vi "Initialize Sensors and Pnuematics.vi"   [LabVIEW 2017]
uses:
  <vilib>/Rock Robotics/SystemInterfaces/AI/FPGA_AIChannel.ctl
  <vilib>/Rock Robotics/SystemInterfaces/DIO/FPGA_DIOChannel.ctl
  <vilib>/Rock Robotics/WPI/Encoder/WPI_EncoderType.ctl
  <vilib>/Rock Robotics/WPI/Solenoid/WPI_SolenoidChannel.ctl
  <vilib>/Rock Robotics/WPI/Utilities/WPI_GetSetVariantRefNum.vi
  Globals/Robot Global Data.vi
  <vilib>/Rock Robotics/WPI/Counter/WPI_CounterDigitalInputToDigitalSource.vi
  <vilib>/Rock Robotics/WPI/Solenoid/WPI_SolenoidOpenSingle.vi
  <vilib>/Rock Robotics/WPI/Switch/WPI_SwitchOpenLimit.vi
types:
  T1 = typedef "WPI_SolenoidChannel.ctl" = enum8{"Solenoid 0", "Solenoid 1", "Solenoid 2", "Solenoid 3", "Solenoid 4", "Solenoid 5", "Solenoid 6", "Solenoid 7", "Invalid"}
  T2 = typedef "WPI_SolenoidDevRef.ctl" = cluster{"DevStatus":errorcluster, "Pneumatics Control Module":u8, "Forward Solenoid Channel":T1, "Reverse Solenoid Channel":T1}
  T3 = typedef "FPGA_DIOChannel.ctl" = enum8{"DIO 0", "DIO 1", "DIO 2", "DIO 3", "DIO 4", "DIO 5", "DIO 6", "DIO 7", "DIO 8", "DIO 9", "DIO MXP 0", "DIO MXP 1", "DIO MXP 2", "DIO MXP 3", "DIO MXP 4", "DIO MXP 5", "DIO MXP 6", "DIO MXP 7", "DIO MXP 8", "DIO MXP 9", "DIO MXP 10", "DIO MXP 11", "DIO MXP 12", "DIO MXP 13", "DIO MXP 14", "DIO MXP 15", "SPI Port CS1", "SPI Port CS2", "SPI Port CS3", "SPI Port MISO", "SPI Port MOSI", "Invalid"}
  T4 = typedef "WPI_EncoderType.ctl" = enum16{"1x", "2x", "4x"}
  T5 = typedef "WPI_DigitalInputDevRef.ctl" = cluster{"DevStatus":errorcluster, "DIO Channel":T3}
  T6 = typedef "FPGA_CounterEncoderSourceConvertionLVSourceType.ctl" = cluster{"DevStatus":errorcluster, "AnalogTriggerMode?":bool, "DigitalMode":cluster{"DIO Channel":T7}, "AnalogTriggerMode":cluster{"AnalogTriggerIndex":T8, "OutputType":T9}}
  T7 = typedef "FPGA_DIODigitalSourceChannel.ctl" = enum8{"DIO 0", "DIO 1", "DIO 2", "DIO 3", "DIO 4", "DIO 5", "DIO 6", "DIO 7", "DIO 8", "DIO 9", "DIO MXP 0", "DIO MXP 1", "DIO MXP 2", "DIO MXP 3", "DIO MXP 4", "DIO MXP 5", "DIO MXP 6", "DIO MXP 7", "DIO MXP 8", "DIO MXP 9", "DIO MXP 10", "DIO MXP 11", "DIO MXP 12", "DIO MXP 13", "DIO MXP 14", "DIO MXP 15", "Disabled"}
  T8 = typedef "FPGA_AnalogTriggerIndex.ctl" = enum8{"Trig 0", "Trig 1", "Trig 2", "Trig 3", "Trig 4", "Trig 5", "Trig 6", "Trig 7", "Invalid"}
  T9 = typedef "FPGA_AnalogTriggerOutType.ctl" = enum16{"InWindow", "TriggerState", "Rising", "Falling"}
  T10 = typedef "WPI_EncoderDevRef.ctl" = cluster{"DevStatus":errorcluster, "EncoderIndex":T11, "CounterIndex":T12, "DistancePerCount":dbl, "Decoding Type":T4}
  T11 = typedef "FPGA_EncoderIdx.ctl" = enum8{"Enc 0", "Enc 1", "Enc 2", "Enc 3", "Enc 4", "Enc 5", "Enc 6", "Enc 7", "Invalid"}
  T12 = typedef "FPGA_CounterCtrSystemIndex.ctl" = enum8{"Ctr 0", "Ctr 1", "Ctr 2", "Ctr 3", "Ctr 4", "Ctr 5", "Ctr 6", "Ctr 7", "Invalid"}
  T13 = typedef "WPI_CompressorDevRef.ctl" = cluster{"DevStatus":errorcluster, "Pneumatics Control Module":u8}
  T14 = typedef "FPGA_AIChannel.ctl" = enum8{"AI 0", "AI 1", "AI 2", "AI 3", "AI MXP 0", "AI MXP 1", "AI MXP 2", "AI MXP 3", "Invalid"}
  T15 = typedef "WPI_AnalogChannelDevRef.ctl" = cluster{"DevStatus":errorcluster, "Analog Channel":T14}
  T16 = typedef "WPI_SwitchDevRef.ctl" = cluster{"DevStatus":errorcluster, "DIO Channel":T3, "CntIndex":T12, "Normally Closed":bool}
  T17 = typedef "WPI_PotentiometerDevRef.ctl" = cluster{"DevStatus":errorcluster, "Analog Channel":T14, "Invert Output":bool}
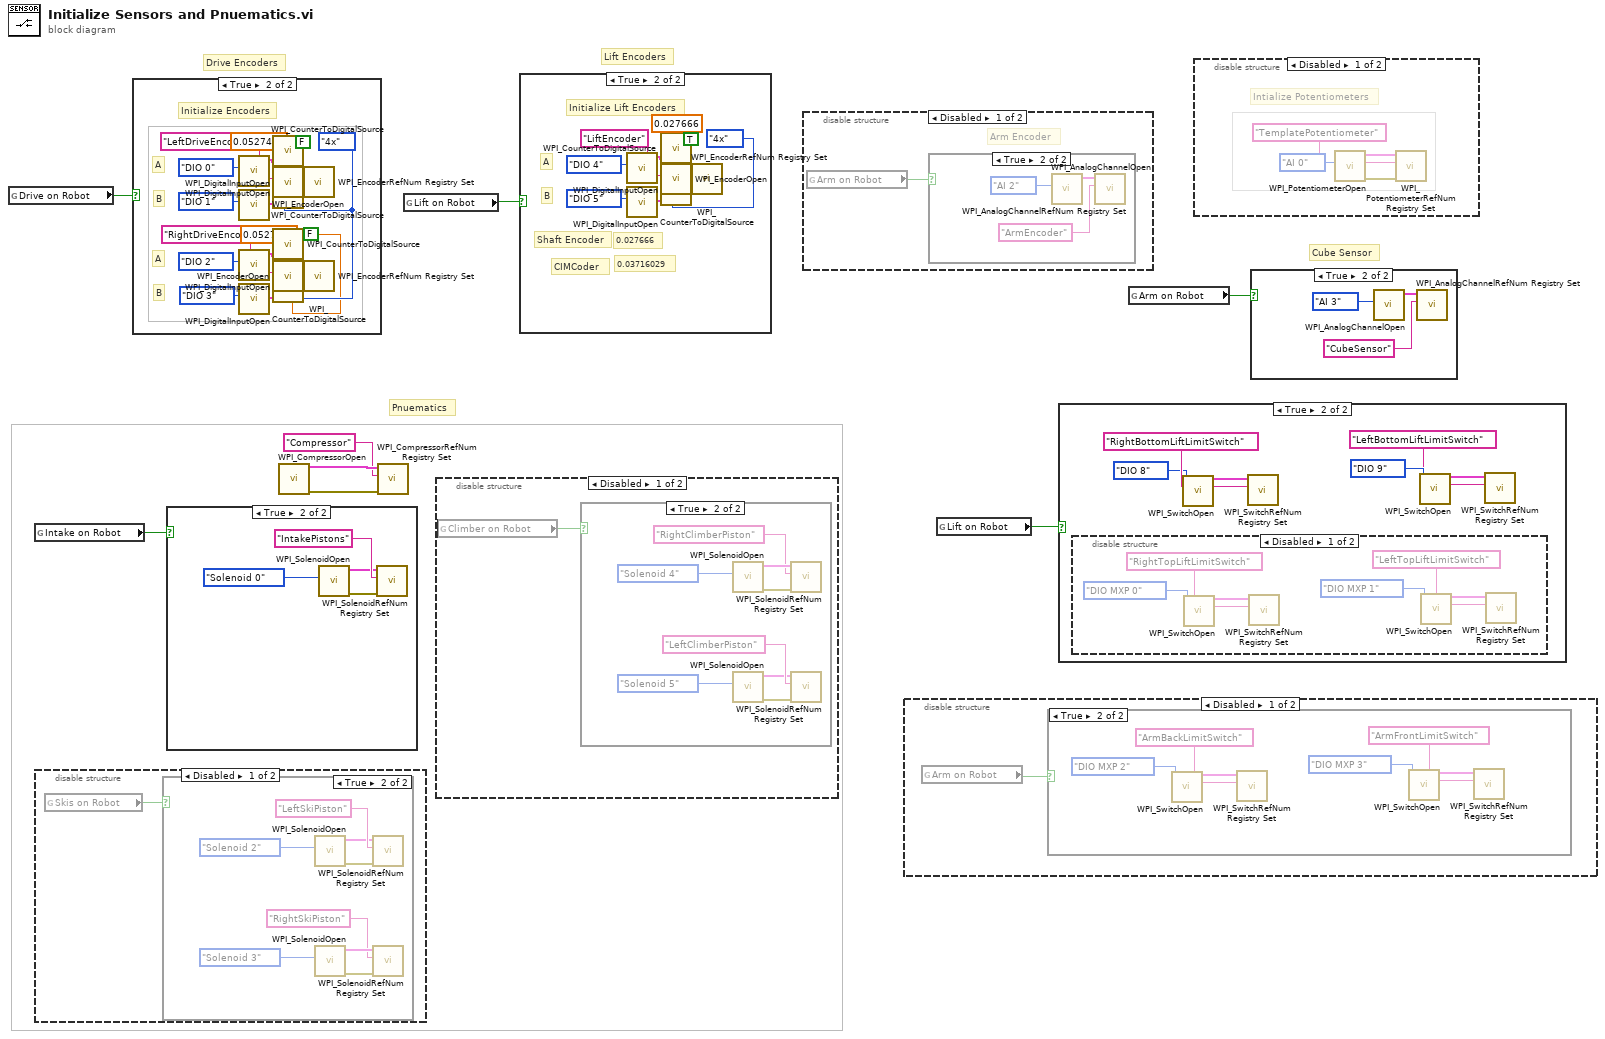
[diagram p0: block diagram]
diagram:
  # "Cube Sensor"
  # "Lift Encoders"
  # "Drive Encoders"
  # "Pnuematics"
  n1 = global read "Robot Global Data.vi" "Drive on Robot"() -> (w5:bool)
  n2 = global read "Robot Global Data.vi" "Intake on Robot"() -> (w4:bool)
  n3 = disable-structure shown="Disabled" {
    frame Disabled {
      n4 = global read "Robot Global Data.vi" "Skis on Robot"() -> (w9:bool)
      n5 = case shown="True" w9 {
        frame False {
        }
        frame True {
          n6 = call-poly <vilib>:"WPI_SolenoidOpen.vi"("Solenoid Channel"=WPI_SolenoidChannel."Solenoid 2") -> ("error out"=w12:errorcluster, "SolenoidDevRef"=w13:T2)  [unwired: 9 in]
          n7 = call-poly <vilib>:"WPI_SolenoidOpen.vi"("Solenoid Channel"=WPI_SolenoidChannel."Solenoid 3") -> ("error out"=w17:errorcluster, "SolenoidDevRef"=w16:T2)  [unwired: 9 in]
          n8 = call <vilib>:"WPI_SolenoidRefNum Registry Set.vi"("error in (no error)"=w12, "refnum name"="LeftSkiPiston", "SolenoidDevRef"=w13) -> ()  [unwired: 7 in, 2 out]
          n9 = call <vilib>:"WPI_SolenoidRefNum Registry Set.vi"("error in (no error)"=w17, "refnum name"="RightSkiPiston", "SolenoidDevRef"=w16) -> ()  [unwired: 7 in, 2 out]
        }
      }
    }
    frame Enabled {
    }
  }
  n10 = case shown="True" w5 {
    frame False {
    }
    frame True {
      w21 = WPI_EncoderType."4x" ("Decoding Type")
      # "B"
      # "A"
      # "B"
      # "A"
      # "Initialize Encoders"
      n11 = call <vilib>:"WPI_DigitalInputOpen.vi"("DIO Channel"=FPGA_DIOChannel."DIO 0") -> ("DigitalInputDevRef"=w38:T5)  [unwired: 1 in, 9 out]
      n12 = call <vilib>:"WPI_DigitalInputOpen.vi"("DIO Channel"=FPGA_DIOChannel."DIO 1") -> ("DigitalInputDevRef"=w39:T5)  [unwired: 1 in, 9 out]
      n13 = call <vilib>:"WPI_DigitalInputOpen.vi"("DIO Channel"=FPGA_DIOChannel."DIO 2") -> ("DigitalInputDevRef"=w29:T5)  [unwired: 1 in, 9 out]
      n14 = call <vilib>:"WPI_DigitalInputOpen.vi"("DIO Channel"=FPGA_DIOChannel."DIO 3") -> ("DigitalInputDevRef"=w30:T5)  [unwired: 1 in, 9 out]
      n15 = call-poly <vilib>:"WPI_CounterToDigitalSource.vi"("DigitalInputDevRef"=w38) -> ("Digital Source"=w37:T6)  [unwired: 6 out]
      n16 = call-poly <vilib>:"WPI_CounterToDigitalSource.vi"("DigitalInputDevRef"=w39) -> ("Digital Source"=w40:T6)  [unwired: 6 out]
      n17 = call <vilib>:"WPI_EncoderOpen.vi"("DistancePerCount"=0.0527473, "Decoding Type"=w21, "Invert Direction (False)"=FALSE, "BSource"=w40, "ASource"=w37) -> ("error out"=w34:errorcluster, "EncoderDevRef"=w33:T10)  [unwired: 3 in, 2 out]
      n18 = call-poly <vilib>:"WPI_CounterToDigitalSource.vi"("DigitalInputDevRef"=w29) -> ("Digital Source"=w28:T6)  [unwired: 6 out]
      n19 = call-poly <vilib>:"WPI_CounterToDigitalSource.vi"("DigitalInputDevRef"=w30) -> ("Digital Source"=w31:T6)  [unwired: 6 out]
      n20 = call <vilib>:"WPI_EncoderOpen.vi"("DistancePerCount"=0.0527473, "Decoding Type"=w21, "Invert Direction (False)"=FALSE, "BSource"=w31, "ASource"=w28) -> ("error out"=w25:errorcluster, "EncoderDevRef"=w24:T10)  [unwired: 3 in, 2 out]
      n21 = call <vilib>:"WPI_EncoderRefNum Registry Set.vi"("error in (no error)"=w34, "refnum name"="LeftDriveEncoder", "EncoderDevRef"=w33) -> ()  [unwired: 7 in, 2 out]
      n22 = call <vilib>:"WPI_EncoderRefNum Registry Set.vi"("error in (no error)"=w25, "refnum name"="RightDriveEncoder", "EncoderDevRef"=w24) -> ()  [unwired: 7 in, 2 out]
    }
  }
  n23 = case shown="True" w4 {
    frame False {
    }
    frame True {
      n24 = call-poly <vilib>:"WPI_SolenoidOpen.vi"("Solenoid Channel"=WPI_SolenoidChannel."Solenoid 0") -> ("error out"=w42:errorcluster, "SolenoidDevRef"=w43:T2)  [unwired: 9 in]
      n25 = call <vilib>:"WPI_SolenoidRefNum Registry Set.vi"("error in (no error)"=w42, "refnum name"="IntakePistons", "SolenoidDevRef"=w43) -> ()  [unwired: 7 in, 2 out]
    }
  }
  n26 = call <vilib>:"WPI_CompressorOpen.vi"() -> ("CompressorDevRef"=w7:T13, "error out"=w8:errorcluster)  [unwired: 14 in]
  n27 = call <vilib>:"WPI_CompressorRefNum Registry Set.vi"("error in (no error)"=w8, "refnum name"="Compressor", "CompressorDevRef"=w7) -> ()  [unwired: 7 in, 2 out]
  n28 = global read "Robot Global Data.vi" "Lift on Robot"() -> (w3:bool)
  n29 = disable-structure shown="Disabled" {
    frame Disabled {
      n30 = global read "Robot Global Data.vi" "Climber on Robot"() -> (w45:bool)
      n31 = case shown="True" w45 {
        frame False {
        }
        frame True {
          n32 = call-poly <vilib>:"WPI_SolenoidOpen.vi"("Solenoid Channel"=WPI_SolenoidChannel."Solenoid 4") -> ("error out"=w53:errorcluster, "SolenoidDevRef"=w52:T2)  [unwired: 9 in]
          n33 = call-poly <vilib>:"WPI_SolenoidOpen.vi"("Solenoid Channel"=WPI_SolenoidChannel."Solenoid 5") -> ("error out"=w48:errorcluster, "SolenoidDevRef"=w49:T2)  [unwired: 9 in]
          n34 = call <vilib>:"WPI_SolenoidRefNum Registry Set.vi"("error in (no error)"=w53, "refnum name"="RightClimberPiston", "SolenoidDevRef"=w52) -> ()  [unwired: 7 in, 2 out]
          n35 = call <vilib>:"WPI_SolenoidRefNum Registry Set.vi"("error in (no error)"=w48, "refnum name"="LeftClimberPiston", "SolenoidDevRef"=w49) -> ()  [unwired: 7 in, 2 out]
        }
      }
    }
    frame Enabled {
    }
  }
  n36 = case shown="True" w3 {
    frame False {
    }
    frame True {
      # "CIMCoder"
      # "Shaft Encoder"
      # "0.03716029"
      # "0.027666"
      # "B"
      # "A"
      # "Initialize Lift Encoders"
      n37 = call <vilib>:"WPI_DigitalInputOpen.vi"("DIO Channel"=FPGA_DIOChannel."DIO 4") -> ("DigitalInputDevRef"=w63:T5)  [unwired: 1 in, 9 out]
      n38 = call <vilib>:"WPI_DigitalInputOpen.vi"("DIO Channel"=FPGA_DIOChannel."DIO 5") -> ("DigitalInputDevRef"=w64:T5)  [unwired: 1 in, 9 out]
      n39 = call-poly <vilib>:"WPI_CounterToDigitalSource.vi"("DigitalInputDevRef"=w63) -> ("Digital Source"=w62:T6)  [unwired: 6 out]
      n40 = call-poly <vilib>:"WPI_CounterToDigitalSource.vi"("DigitalInputDevRef"=w64) -> ("Digital Source"=w65:T6)  [unwired: 6 out]
      n41 = call <vilib>:"WPI_EncoderOpen.vi"("DistancePerCount"=0.027666, "Decoding Type"=WPI_EncoderType."4x", "Invert Direction (False)"=TRUE, "BSource"=w65, "ASource"=w62) -> ("error out"=w59:errorcluster, "EncoderDevRef"=w58:T10)  [unwired: 3 in, 2 out]
      n42 = call <vilib>:"WPI_EncoderRefNum Registry Set.vi"("error in (no error)"=w59, "refnum name"="LiftEncoder", "EncoderDevRef"=w58) -> ()  [unwired: 7 in, 2 out]
    }
  }
  n43 = disable-structure shown="Disabled" {
    frame Disabled {
      # "Arm Encoder"
      n44 = global read "Robot Global Data.vi" "Arm on Robot"() -> (w66:bool)
      n45 = case shown="True" w66 {
        frame False {
        }
        frame True {
          n46 = call <vilib>:"WPI_AnalogChannelOpen.vi"("Analog Channel"=FPGA_AIChannel."AI 2") -> ("AIDeviceRef"=w68:T15)  [unwired: 9 in, 1 out]
          n47 = call <vilib>:"WPI_AnalogChannelRefNum Registry Set.vi"("refnum name"="ArmEncoder", "AIDeviceRef"=w68) -> ()  [unwired: 8 in, 2 out]
        }
      }
    }
    frame Enabled {
    }
  }
  n48 = disable-structure shown="Disabled" {
    frame Disabled {
      n49 = global read "Robot Global Data.vi" "Arm on Robot"() -> (w70:bool)
      n50 = case shown="True" w70 {
        frame False {
        }
        frame True {
          n51 = call-poly <vilib>:"WPI_SwitchOpen.vi"("DIO Channel"=FPGA_DIOChannel."DIO MXP 2") -> ("SwitchDevRef"=w76:T16)  [unwired: 9 in, 1 out]
          n52 = call <vilib>:"WPI_SwitchRefNum Registry Set.vi"("refnum name"="ArmBackLimitSwitch", "SwitchDevRef"=w76) -> ()  [unwired: 8 in, 2 out]
          n53 = call-poly <vilib>:"WPI_SwitchOpen.vi"("DIO Channel"=FPGA_DIOChannel."DIO MXP 3") -> ("SwitchDevRef"=w71:T16)  [unwired: 9 in, 1 out]
          n54 = call <vilib>:"WPI_SwitchRefNum Registry Set.vi"("refnum name"="ArmFrontLimitSwitch", "SwitchDevRef"=w71) -> ()  [unwired: 8 in, 2 out]
        }
      }
    }
    frame Enabled {
    }
  }
  n55 = global read "Robot Global Data.vi" "Lift on Robot"() -> (w2:bool)
  n56 = case shown="True" w2 {
    frame False {
    }
    frame True {
      n57 = disable-structure shown="Disabled" {
        frame Disabled {
          n58 = call-poly <vilib>:"WPI_SwitchOpen.vi"("DIO Channel"=FPGA_DIOChannel."DIO MXP 0") -> ("SwitchDevRef"=w83:T16)  [unwired: 9 in, 1 out]
          n59 = call <vilib>:"WPI_SwitchRefNum Registry Set.vi"("refnum name"="RightTopLiftLimitSwitch", "SwitchDevRef"=w83) -> ()  [unwired: 8 in, 2 out]
          n60 = call-poly <vilib>:"WPI_SwitchOpen.vi"("DIO Channel"=FPGA_DIOChannel."DIO MXP 1") -> ("SwitchDevRef"=w88:T16)  [unwired: 9 in, 1 out]
          n61 = call <vilib>:"WPI_SwitchRefNum Registry Set.vi"("refnum name"="LeftTopLiftLimitSwitch", "SwitchDevRef"=w88) -> ()  [unwired: 8 in, 2 out]
        }
        frame Enabled {
        }
      }
      n62 = call-poly <vilib>:"WPI_SwitchOpen.vi"("DIO Channel"=FPGA_DIOChannel."DIO 8") -> ("SwitchDevRef"=w82:T16)  [unwired: 9 in, 1 out]
      n63 = call <vilib>:"WPI_SwitchRefNum Registry Set.vi"("refnum name"="RightBottomLiftLimitSwitch", "SwitchDevRef"=w82) -> ()  [unwired: 8 in, 2 out]
      n64 = call-poly <vilib>:"WPI_SwitchOpen.vi"("DIO Channel"=FPGA_DIOChannel."DIO 9") -> ("SwitchDevRef"=w77:T16)  [unwired: 9 in, 1 out]
      n65 = call <vilib>:"WPI_SwitchRefNum Registry Set.vi"("refnum name"="LeftBottomLiftLimitSwitch", "SwitchDevRef"=w77) -> ()  [unwired: 8 in, 2 out]
    }
  }
  n66 = global read "Robot Global Data.vi" "Arm on Robot"() -> (w1:bool)
  n67 = disable-structure shown="Disabled" {
    frame Disabled {
      # "Intialize Potentiometers"
      n68 = call <vilib>:"WPI_PotentiometerOpen.vi"("Analog Channel"=FPGA_AIChannel."AI 0") -> ("error out"=w91:errorcluster, "PotDevRef"=w90:T17)  [unwired: 9 in]
      n69 = call <vilib>:"WPI_PotentiometerRefNum Registry Set.vi"("error in (no error)"=w91, "refnum name"="TemplatePotentiometer", "PotDevRef"=w90) -> ()  [unwired: 7 in, 2 out]
    }
    frame Enabled {
    }
  }
  n70 = case shown="True" w1 {
    frame False {
    }
    frame True {
      n71 = call <vilib>:"WPI_AnalogChannelOpen.vi"("Analog Channel"=FPGA_AIChannel."AI 3") -> ("AIDeviceRef"=w94:T15)  [unwired: 9 in, 1 out]
      n72 = call <vilib>:"WPI_AnalogChannelRefNum Registry Set.vi"("refnum name"="CubeSensor", "AIDeviceRef"=w94) -> ()  [unwired: 8 in, 2 out]
    }
  }
